vi "Msg.vi"(7 "jettl in":refnum<class "jettl.lvclass">, 11 "Pop Up Msg Strategy in":refnum<class "Pop Up Msg Strategy.lvclass">) -> (5 "jettl out":refnum<class "jettl.lvclass">)   [LabVIEW 2021, in "jettl Msg Pop Up.lvlib" / "Pop Up Msg Strategy.lvclass"]
uses:
  Pop Up Msg Strategy.lvclass
  jettl/jettl/jettl.lvclass
  Pop Up/Pop Up.lvclass
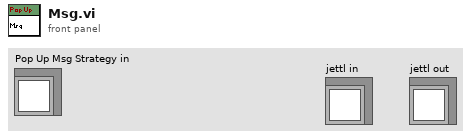
[diagram p1: front panel]
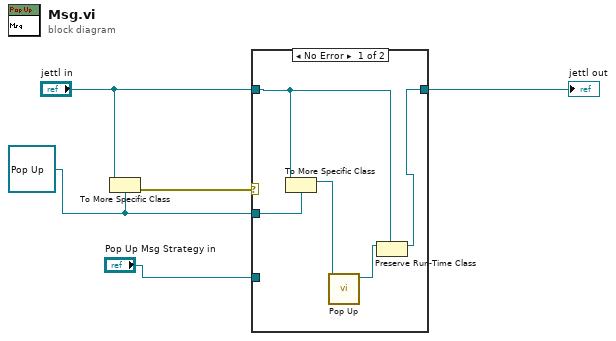
[diagram p0: block diagram]
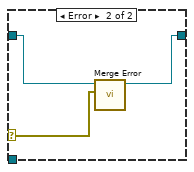
[diagram p2: hidden frame]
diagram:
  w3 = refnum<class "Pop Up.lvclass"> refnum ("Pop Up.lvlib:Pop Up.lvclass")
  n1 = To More Specific Class(target class=w3, reference="jettl in") -> (error out=w5:errorcluster)  [unwired: 1 in, 1 out]
  n2 = case shown="No Error" w5 {
    selector: w5 -> [_ w13]
    tunnel: [w6 w11] -> w1
    tunnel: "jettl in" -> [w8 w12]
    tunnel: w3 -> [w10 _]
    tunnel: "Pop Up Msg Strategy in" -> [_ _]
    frame No Error {
      n3 = To More Specific Class(target class=w10, reference=w8) -> (specific class reference=w9:refnum<class "Pop Up.lvclass">)  [unwired: 1 in, 1 out]
      n4 = call-dynamic "Pop Up.vi"("Pop Up in"=w9) -> ("Pop Up out"=w7:refnum<class "Pop Up.lvclass">)  [unwired: 10 in]
      n5 = Preserve Run-Time Class(object in=w7, 2:w8) -> (object out=w6:refnum<class "jettl.lvclass">)  [unwired: 1 in, 1 out]
    }
    frame Error {
      n6 = call-dynamic "Merge Error.vi"("Error"=w13, "Merge Error in"=w12) -> ("Merge Error out"=w11:refnum<class "jettl.lvclass">)  [unwired: 9 in]
    }
  }
  "jettl out" <- w1
